vi "libssh2_knownhost_readfile.vi"(8 "error in (no error)":errorcluster, 9 "type":i32, 10 "filename":string, 11 "Hosts":T1) -> (0 "error out":errorcluster, 3 "return value":i32)   [LabVIEW 2013, in "libssh2.lvlib"]
uses:
  libssh2.lvlib
  Hosts Refnum.ctl
  libssh2.dll
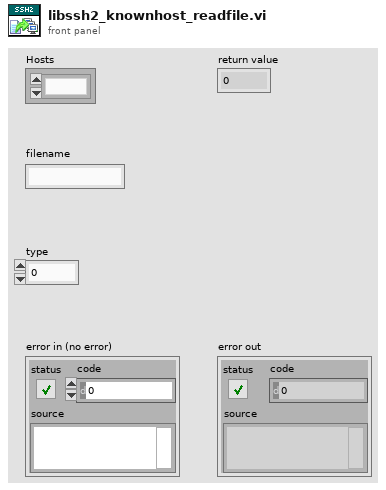
[diagram p1: front panel]
types:
  T1 = typedef "libssh2.lvlib/Hosts Refnum.ctl" = refnum<k1>
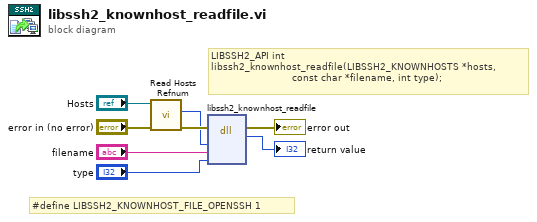
[diagram p0: block diagram]
diagram:
  # "#define LIBSSH2_KNOWNHOST_FILE_OPENSSH 1"
  # "LIBSSH2_API int\nlibssh2_knownhost_readfile(LIBSSH2_KNOWNHOSTS *hosts,\n                           const char *filename, int type);"
  n1 = call "Read Hosts Refnum.vi"("error in (no error)"="error in (no error)", "Hosts"="Hosts") -> ("error out"=w3:errorcluster, "LIBSSH2_KNOWNHOSTS*"=w1:u64)  [unwired: 8 in]
  n2 = dll-call lib="C:/Users/pasca/source/repos/libssh2-labview/libssh2**.*" fn="libssh2_knownhost_readfile"(error in=w3, "hosts"=w1, "filename"="filename", "type"="type") -> (error out=→"error out":errorcluster, "return value"=→"return value":i32)  [unwired: 5 in, 1 out]
